vi "control loop update execution timing tags.vi"(9 "execution timing in":T2, 10 "execution inidces in":T1, 11 "control loop data in":T3) -> (1 "execution timing out":T2, 2 "execution inidces out":T1, 3 "control loop data out":T3)   [LabVIEW 2013, in "main engine.lvlib"]
doc: "This VI can be used to write any engine-relate metrics required before the current cycle's module execution begins."
uses:
  main engine.lvlib
  control loop data.ctl
  <vilib>/NI/Tag Bus/table/data table.ctl
  engine run schedule.ctl
  engine decimation schedule.ctl
  full module data.ctl
  <vilib>/NI/Tag Bus Module Framework/runtime/TBM module execution interface.lvclass
  module run state.ctl
  async executor/asynchronous executor reference.ctl
  async executor/async message to executor.ctl
  Runtime/async command notification.ctl
  Runtime/async error info.ctl
  <vilib>/NI/Tag Bus Module Framework/runtime/error classification.ctl
  <vilib>/NI/Tag Bus Module Framework/module configuration/TBM module configuration.lvclass
  module method data.ctl
  <vilib>/NI/Tag Bus/table/transfer specification.ctl
  <vilib>/NI/Tag Bus/tag/Data Type.ctl
  fault handling spec.ctl
  Configuration/Error Actions.ctl
  execution timing indices.ctl
  execution times.ctl
  <vilib>/NI/Tag Bus/table/data polymorphs/write one/write Double.vi
  <vilib>/NI/Tag Bus/table/data table.lvlib
  <vilib>/NI/Tag Bus/tag/tag descriptor.lvclass
  Configuration/Standard Engine Configuration.lvclass
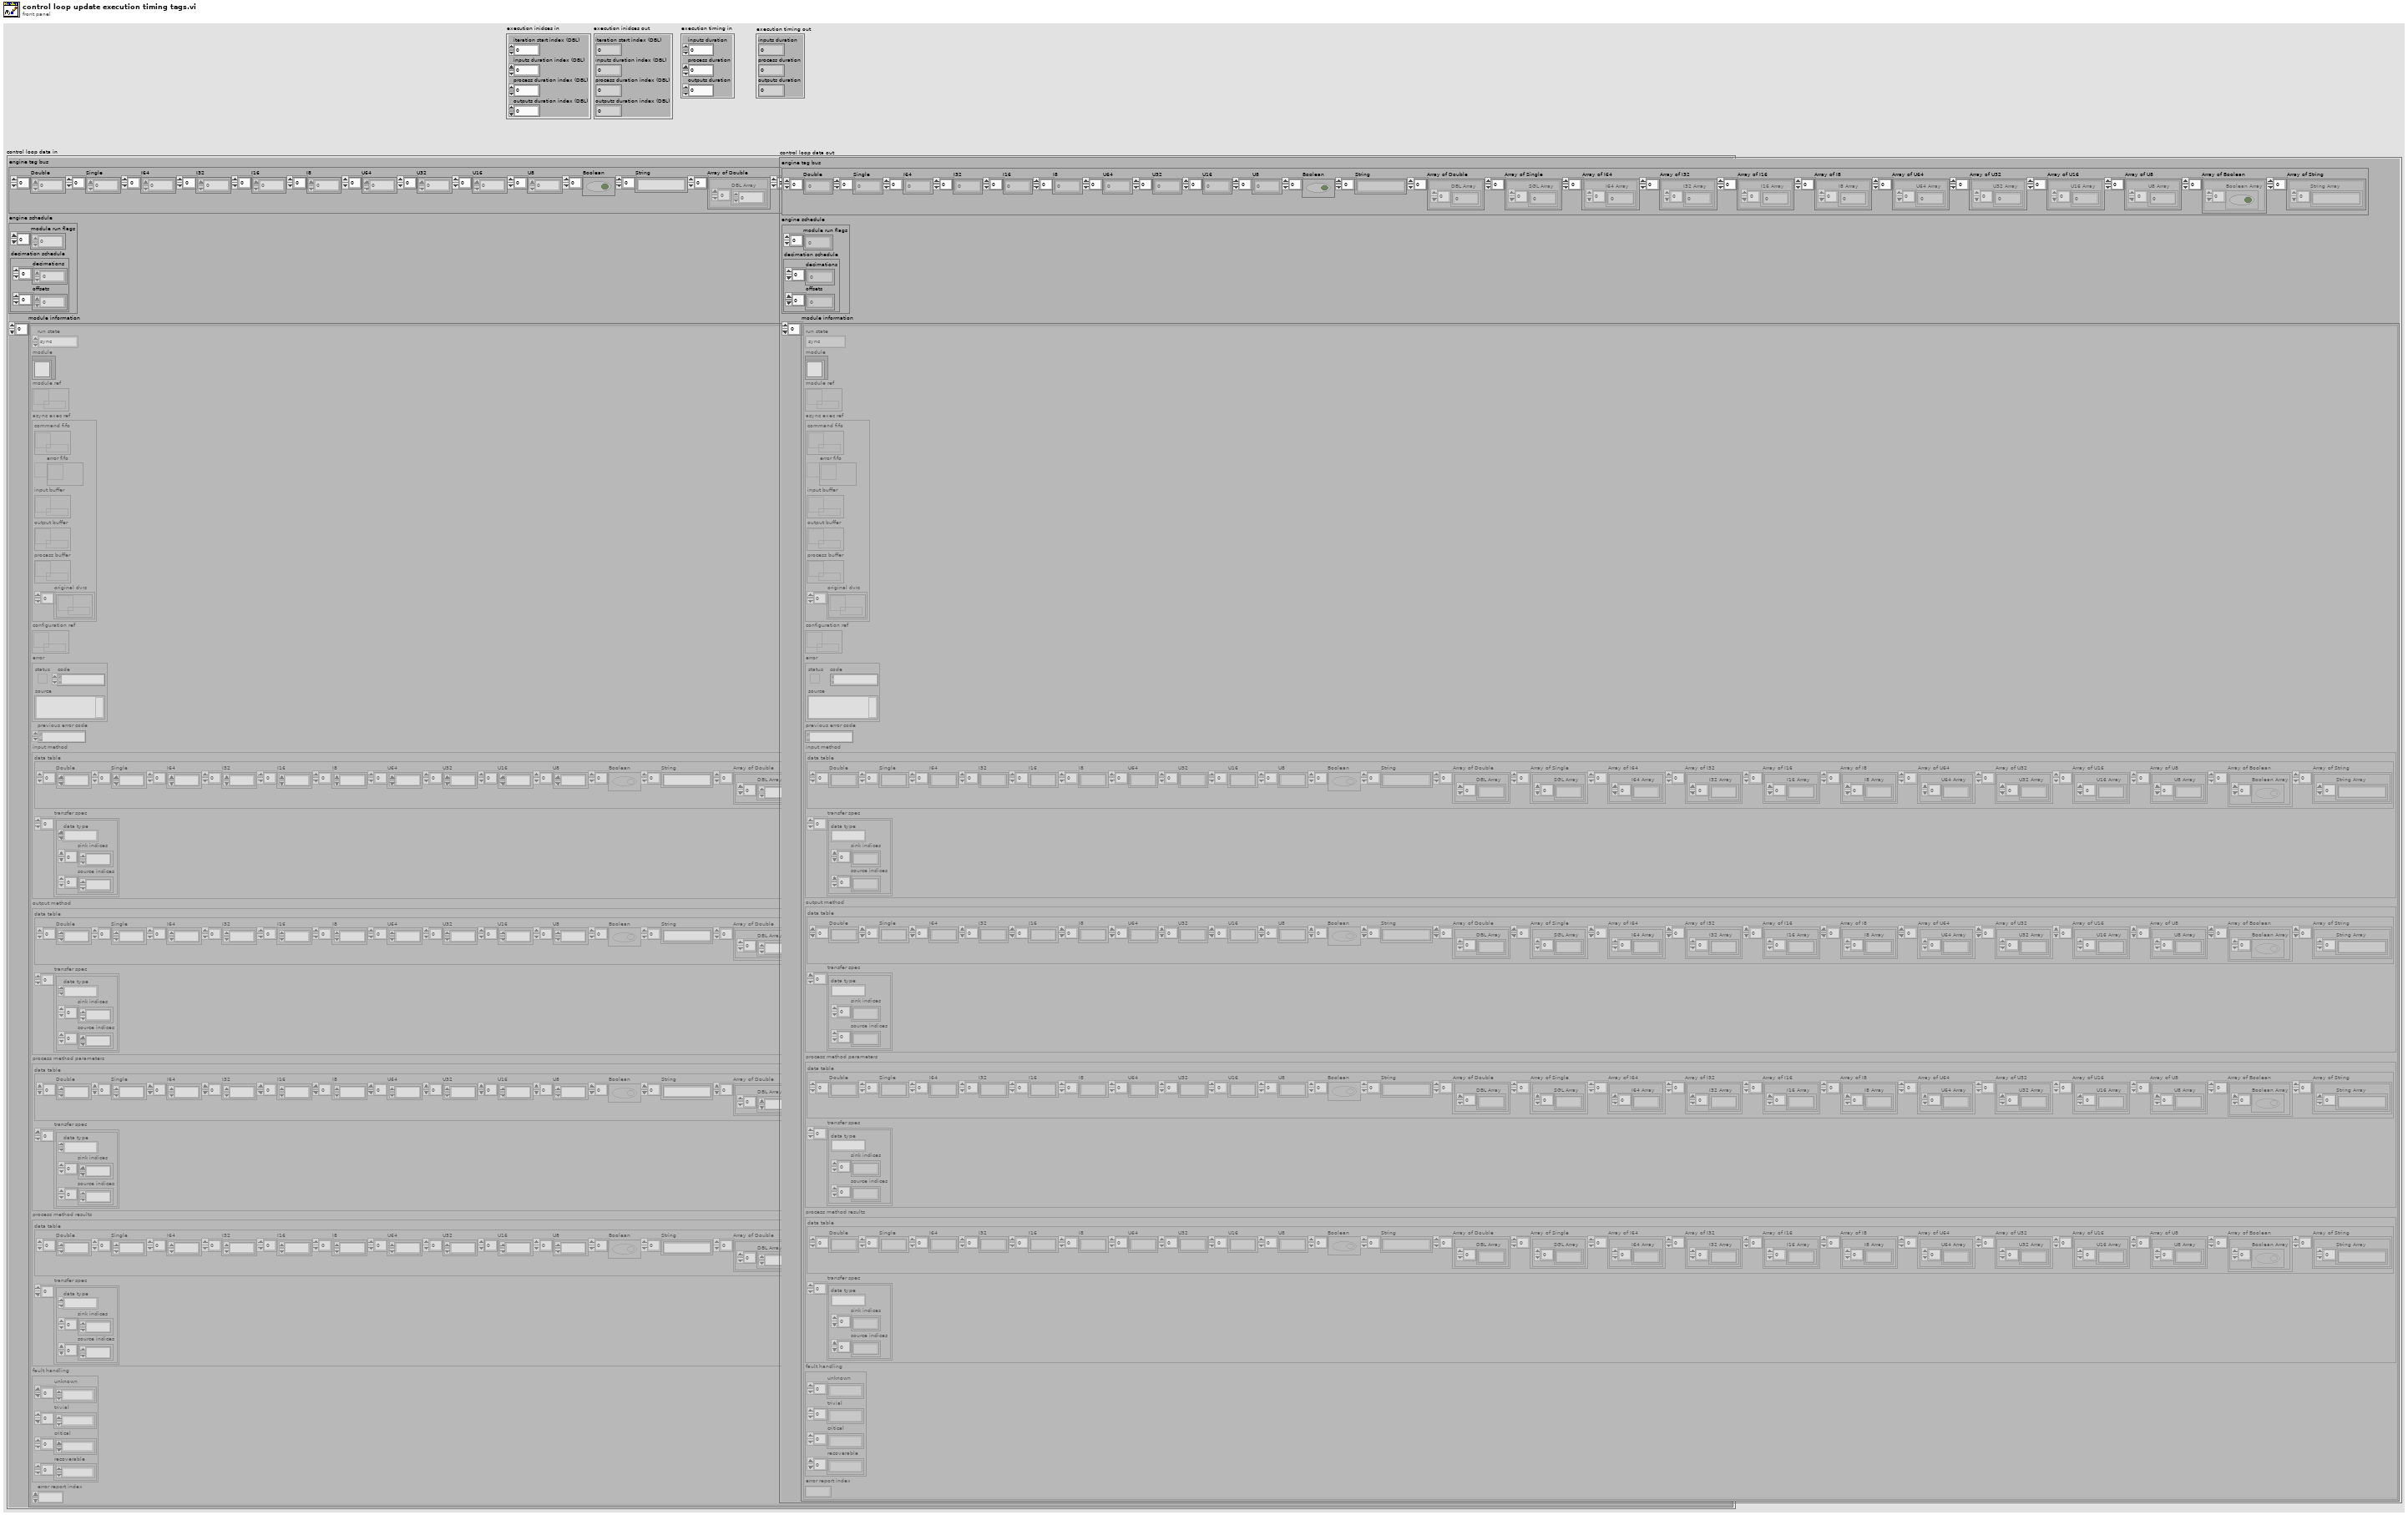
[diagram p1: front panel]
types:
  T1 = typedef "main engine.lvlib/execution timing indices.ctl" = cluster{"iteration start index (DBL)":i32, "inputs duration index (DBL)":i32, "process duration index (DBL)":i32, "outputs duration index (DBL)":i32}
  T2 = typedef "main engine.lvlib/execution times.ctl" = cluster{"inputs duration":dbl, "process duration":dbl, "outputs duration":dbl}
  T3 = typedef "main engine.lvlib/control loop data.ctl" = cluster{"engine tag bus":T4, "engine schedule":T5, "module information":T7[]}
  T4 = typedef "tag bus.lvlib/data table.lvlib/data table.ctl" = cluster{"Double":dbl[], "Single":sgl[], "I64":i64[], "I32":i32[], "I16":i16[], "I8":i8[], "U64":u64[], "U32":u32[], "U16":u16[], "U8":u8[], "Boolean":bool[], "String":string[], "Array of Double":cluster{"DBL Array":dbl[]}[], "Array of Single":cluster{"SGL Array":sgl[]}[], "Array of I64":cluster{"I64 Array":i64[]}[], "Array of I32":cluster{"I32 Array":i32[]}[], "Array of I16":cluster{"I16 Array":i16[]}[], "Array of I8":cluster{"I8 Array":i8[]}[], "Array of U64":cluster{"U64 Array":u64[]}[], "Array of U32":cluster{"U32 Array":u32[]}[], "Array of U16":cluster{"U16 Array":u16[]}[], "Array of U8":cluster{"U8 Array":u8[]}[], "Array of Boolean":cluster{"Boolean Array":bool[]}[], "Array of String":cluster{"String Array":string[]}[]}
  T5 = typedef "main engine.lvlib/engine run schedule.ctl" = cluster{"module run flags":u8[], "decimation schedule":T6}
  T6 = typedef "main engine.lvlib/engine decimation schedule.ctl" = cluster{"decimations":u16[], "offsets":u16[]}
  T7 = typedef "main engine.lvlib/full module data.ctl" = cluster{"run state":T8, "module":refnum<class "TBM module execution interface.lvclass">, "module ref":refnum<data-value>, "async exec ref":T9, "configuration ref":refnum<data-value>, "error":errorcluster, "previous error code":i32, "input method":T10, "output method":T10, "process method parameters":T10, "process method results":T10, "fault handling":T13, "error report index ":i32}
  T8 = typedef "main engine.lvlib/module run state.ctl" = enum16{"sync", "async"}
  T9 = typedef "main engine.lvlib/asynchronous executor reference.ctl" = cluster{"command fifo":refnum<k33>, "error fifo":refnum<k33>, "input buffer":refnum<k33>, "output buffer":refnum<k33>, "process buffer":refnum<k33>, "original dvrs":refnum<data-value>[]}
  T10 = typedef "main engine.lvlib/module method data.ctl" = cluster{"data table":T4, "transfer spec":T11[]}
  T11 = typedef "tag bus.lvlib/data table.lvlib/transfer specification.ctl" = cluster{"data type":T12, "sink indices":i32[], "source indices":i32[]}
  T12 = typedef "tag bus.lvlib/tag descriptor.lvclass/Data Type.ctl" = enum16{"Double", "Single", "I64", "I32", "I16", "I8", "U64", "U32", "U16", "U8", "Boolean", "String", "Array of Double", "Array of Single", "Array of I64", "Array of I32", "Array of I16", "Array of I8", "Array of U64", "Array of U32", "Array of U16", "Array of U8", "Array of Boolean", "Array of String"}
  T13 = typedef "main engine.lvlib/fault handling spec.ctl" = cluster{"unknown":T14[], "trivial":T14[], "critical":T14[], "recoverable":T14[]}
  T14 = typedef "Standard Engine Configuration.lvclass/Error Actions.ctl" = enum16{"Clear", "Notify", "Log", "Stop Component", "Stop Engine", "Safe State", "Attempt Recovery"}
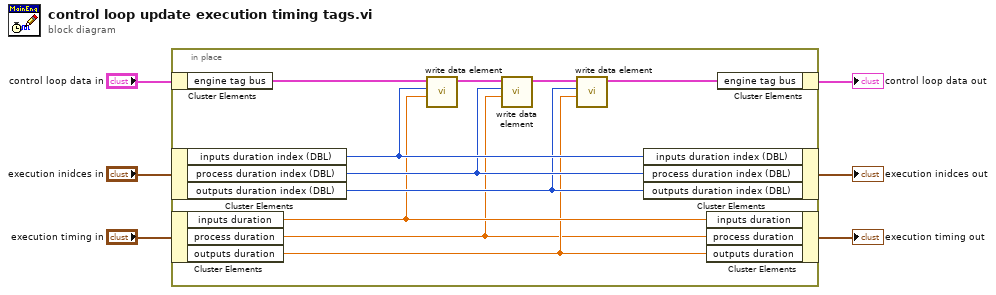
[diagram p0: block diagram]
diagram:
  n1 = in-place {
    n2 = in-place-cluster #1("control loop data in") -> ("engine tag bus"=w16:T4)
    n3 = in-place-cluster #2("execution inidces in") -> ("inputs duration index (DBL)"=w12:i32, "process duration index (DBL)"=w11:i32, "outputs duration index (DBL)"=w10:i32)
    n4 = in-place-cluster #3("execution timing in") -> ("inputs duration"=w9:dbl, "process duration"=w7:dbl, "outputs duration"=w8:dbl)
    n5 = call-poly <vilib>:"write data element.vi"("value"=w9, "index"=w12, "data table in"=w16) -> ("data table out"=w15:T4)  [unwired: 8 in]
    n6 = call-poly <vilib>:"write data element.vi"("value"=w7, "index"=w11, "data table in"=w15) -> ("data table out"=w13:T4)  [unwired: 8 in]
    n7 = call-poly <vilib>:"write data element.vi"("value"=w8, "index"=w10, "data table in"=w13) -> ("data table out"=w14:T4)  [unwired: 8 in]
    n8 = in-place-cluster #2("inputs duration index (DBL)"=w12, "process duration index (DBL)"=w11, "outputs duration index (DBL)"=w10) -> (→"execution inidces out":T1)
    n9 = in-place-cluster #3("inputs duration"=w9, "process duration"=w7, "outputs duration"=w8) -> (→"execution timing out":T2)
    n10 = in-place-cluster #1("engine tag bus"=w14) -> (→"control loop data out":T3)
  }
